vi "Test Server (Dan King's conflicted copy 2015-11-25).vi"() -> ()   [LabVIEW 2015, in "Test EMS.lvlib"]
doc: "This example shows how to set status values of <b>DPS</b> points with IEC61850 MMS server VIs.\n\nWhile this VI is running, an IEC61850 MMS server is available. Use corresponding clients to connect to this server and read these ST values. You can change the <b>DPS</b> Status while the VI is running. If you change the <b>DPS</b> Status, the values that the clients read from the server also change."
uses:
  Test EMS.lvlib
  <vilib>/Modbus/slave/Create Slave Instance (TCP).vi
  <vilib>/Modbus/slave/Modbus Slave.lvclass
panel:
  in  "stop":bool
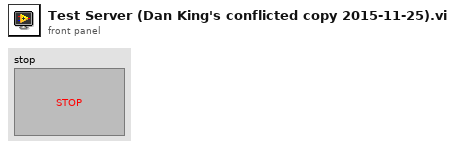
[diagram p1: front panel]
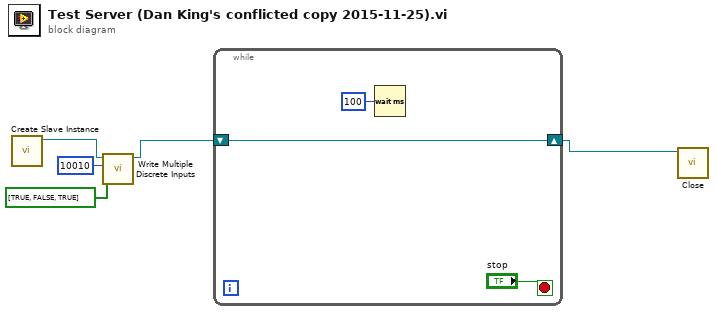
[diagram p0: block diagram]
diagram:
  n1 = call-poly <vilib>:"Create Slave Instance.vi"() -> ("TCP slave instance"=w3:refnum<class "Modbus Slave.lvclass">)  [unwired: 10 in, 1 out]
  n2 = call-dynamic "Write Multiple Discrete Inputs.vi"("discrete input values"=bool[] [TRUE, FALSE, TRUE], "starting address"=u16 10010, "Modbus slave in"=w3) -> ("Modbus slave out"=w5:refnum<class "Modbus Slave.lvclass">)  [unwired: 7 in, 1 out]
  n3 = while {
    shift-right: [w8] -> w4
    shift-left: w5 -> [w8]
    stop <- "stop" stop-if-true
    n4 = Wait (ms)(milliseconds to wait=u32 100) -> ()  [unwired: 1 out]
  }
  n5 = call-dynamic "Close.vi"("Modbus slave in"=w4) -> ()  [unwired: 10 in, 1 out]
